vi "Query Time Format.vi"(8 "error IO":errorcluster, 11 "VISA resource name":refnum<visa-resource-name>) -> (0 "error Out":errorcluster, 2 "Time Format":enum16{"12hr", "24hr"}(ring), 3 "VISA resource Out":refnum<visa-resource-name>)   [LabVIEW 2020, in "eec EST 300.lvlib"]
doc: "STF?\nReturns the status of the clock format. 12 hour or 24 hour."
uses:
  <instrlib>/eec EST 300/eec EST 300.lvlib
panel:
  # "0 - 12 hr\n1 - 24 hr"
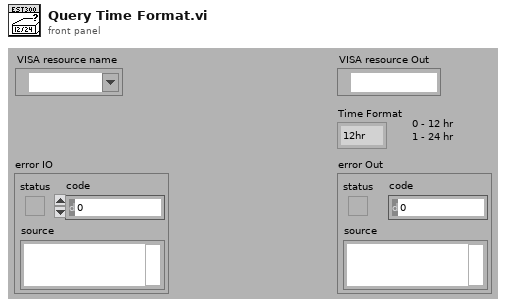
[diagram p1: front panel]
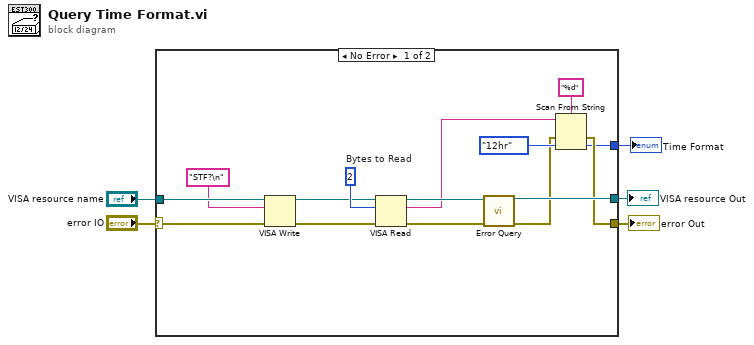
[diagram p0: block diagram]
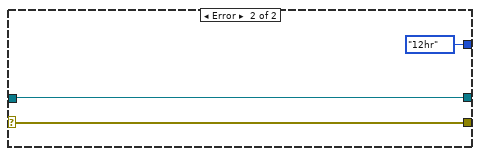
[diagram p2: hidden frame]
diagram:
  n1 = case shown="No Error" "error IO" {
    selector: "error IO" -> [w20 w23]
    tunnel: [w7 w23] -> w2
    tunnel: [w18 w22] -> w3
    tunnel: "VISA resource name" -> [w19 w22]
    tunnel: [w6 enum16{"12hr", "24hr"}."12hr" ("Time Format")] -> w1
    frame No Error {
      w14 = u32 2  # Bytes to Read
      n2 = VISA Write(VISA resource name=w19, write buffer="STF?\n" ("Command to Send (empty)"), error in (no error)=w20) -> (VISA resource name out=w13:refnum<visa-resource-name>, error out=w12:errorcluster)  [unwired: 1 out]
      n3 = VISA Read(VISA resource name=w13, byte count=w14, error in (no error)=w12) -> (VISA resource name out=w16:refnum<visa-resource-name>, read buffer=w10:string, error out=w15:errorcluster)  [unwired: 1 out]
      n4 = call <instrlib>:"Error Query.vi"("VISA resource name"=w16, "error in (no error)"=w15) -> ("VISA resource name out"=w18:refnum<visa-resource-name>, "error out"=w8:errorcluster)  [unwired: 10 in, 2 out]
      n5 = Scan From String(format string="%d", input string=w10, error in=w8, default 1=enum16{"12hr", "24hr"}."12hr" ("Time Format")) -> (error out=w7:errorcluster, output 1=w6:enum16{"12hr", "24hr"})  [unwired: 1 in, 2 out]
    }
    frame Error {
    }
  }
  "VISA resource Out" <- w3
  "error Out" <- w2
  "Time Format" <- w1
